vi "DELETE.vi"() -> ()   [LabVIEW 2024]
uses:
  <vilib>/addons/database/Connection.llb/Conn ObjectReference.ctl
  <vilib>/addons/database/NI_Database_API.lvlib
panel:
  in  "input 1":string
  in  "Boolean":bool
  out "connection reference 2":T1
  in  "connection reference":T1
  out "error out":errorcluster
  in  "error in (no error)":errorcluster
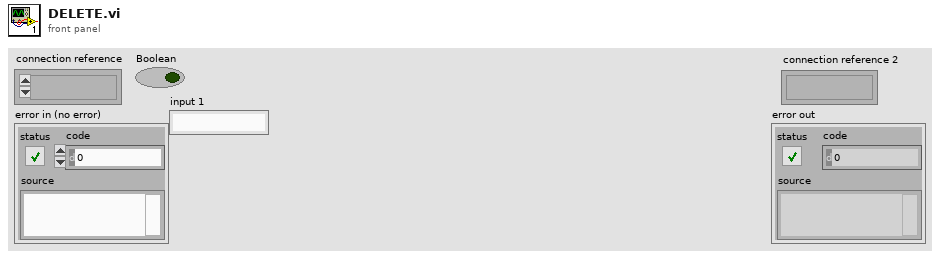
[diagram p1: front panel]
types:
  T1 = typedef "NI_Database_API.lvlib/Conn ObjectReference.ctl" = refnum<k1>
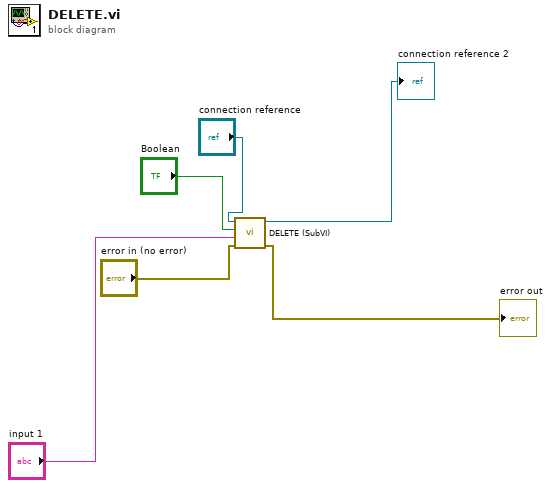
[diagram p0: block diagram]
diagram:
  n1 = call "DELETE (SubVI).vi"("error in (no error)"="error in (no error)", "input 1"="input 1", "Boolean"="Boolean", "Refnum in"="connection reference") -> ("error out"=→"error out":errorcluster, "Refnum out"=→"connection reference 2":T1)  [unwired: 6 in]
